vi "CheckDriveStatus.vi"(2 "Channel Properties":T1={"Channel Name"="", "Vel. Default"=5.0, "Acc. Default"=5.0, "Vel. Max"=5.0, "Vel. Min"=5.0, "Acc. Max"=5.0, "Acc. Min"=5.0, "Pulses/unit"=0.0, "Address"=0, "Pulse Offset"=0, "Pos Tolerance"=0.0, "Pulses/rev"=0.0, "Backlash/Eng units"=0.0, "Current Pos"=0.0, "Ch Status"=enum."Active", "Port Name"="", "Axis Transform mode"="", "Metadata Ch Name"="", "Type"=""} {"Current Pos" format="%.2f"; "Backlash/Eng units" format="%.2f"; "Pulses/rev" format="%.2f"; "Pos Tolerance" format="%.2f"; "Pulses/unit" format="%.2f"; "Acc. Min" format="%.2f"; "Acc. Max" format="%.2f"; "Vel. Min" format="%.2f"; "Vel. Max" format="%.2f"; "Acc. Default" format="%.2f"; "Vel. Default" format="%.2f"}, 3 "Axis info cluster":T2) -> (0 "Error string":string, 1 "Axis info cluster Out":T2)   [LabVIEW 2012]
uses:
  DriveStatus.ctl
  DriveProperties.ctl
  GenericDriveCommand.ctl
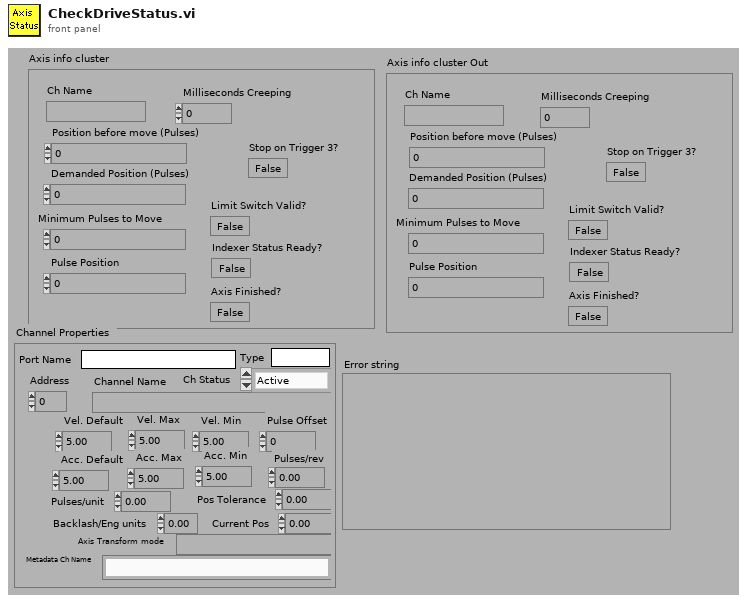
[diagram p1: front panel]
types:
  T1 = typedef "DriveProperties.ctl" = cluster{"Channel Name":string, "Vel. Default":dbl, "Acc. Default":dbl, "Vel. Max":dbl, "Vel. Min":dbl, "Acc. Max":dbl, "Acc. Min":dbl, "Pulses/unit":dbl, "Address":u8, "Pulse Offset":i32, "Pos Tolerance":dbl, "Pulses/rev":dbl, "Backlash/Eng units":dbl, "Current Pos":dbl, "Ch Status":enum16{"Active", "Offline", "Simulate"}, "Port Name":string, "Axis Transform mode":string, "Metadata Ch Name":string, "Type":string}
  T2 = typedef "DriveStatus.ctl" = cluster{"Ch Name":string, "Position before move (Pulses)":dbl, "Demanded Position (Pulses)":dbl, "Minimum Pulses to Move":dbl, "Pulse Position":dbl, "Indexer Status Ready?":bool, "Axis Finished?":bool, "Limit Switch Valid?":bool, "Milliseconds Creeping":u32, "Stop on Trigger 3?":bool}
  T3 = typedef "GenericDriveCommand.ctl" = string
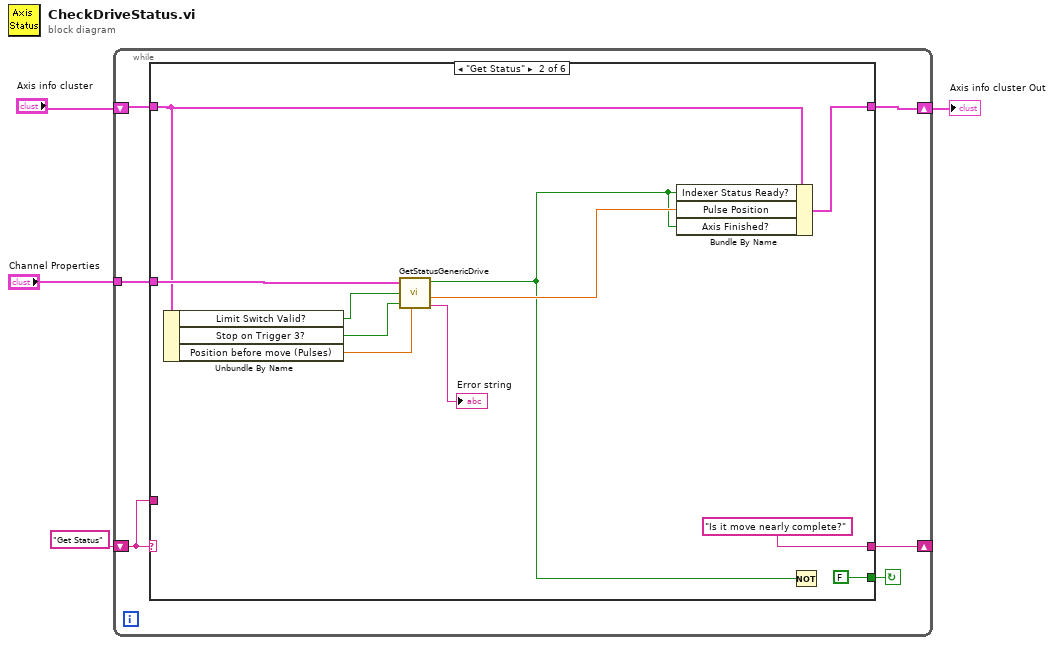
[diagram p0: block diagram]
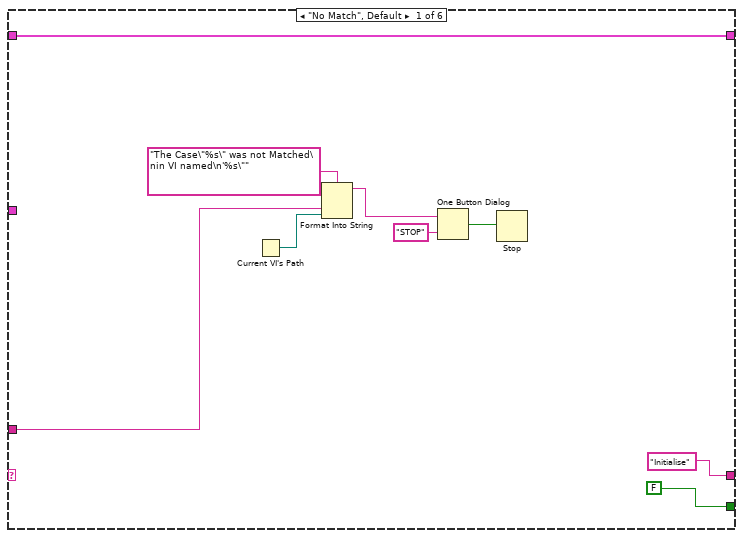
[diagram p2: hidden frame]
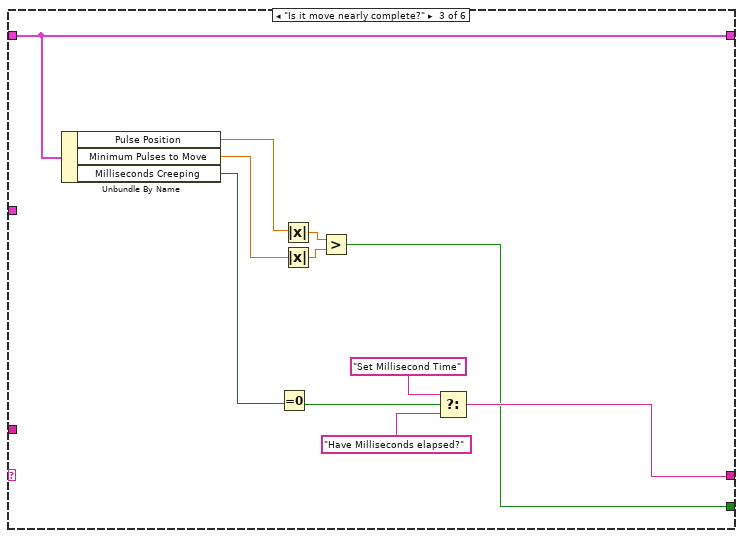
[diagram p3: hidden frame]
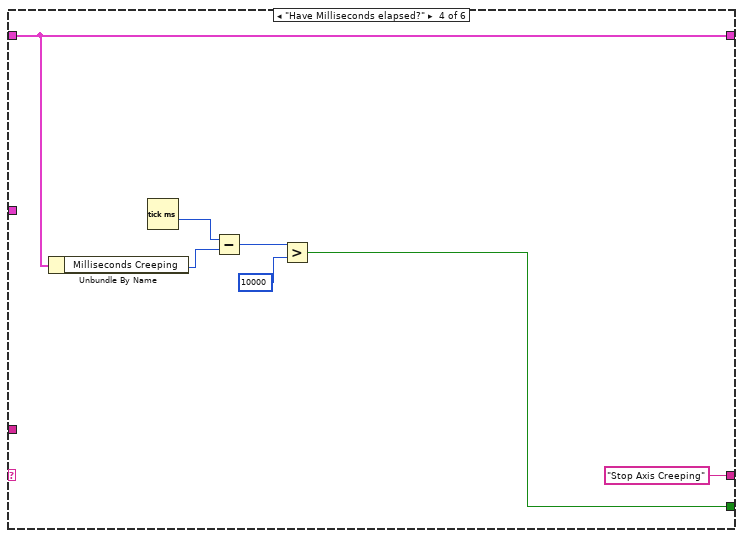
[diagram p4: hidden frame]
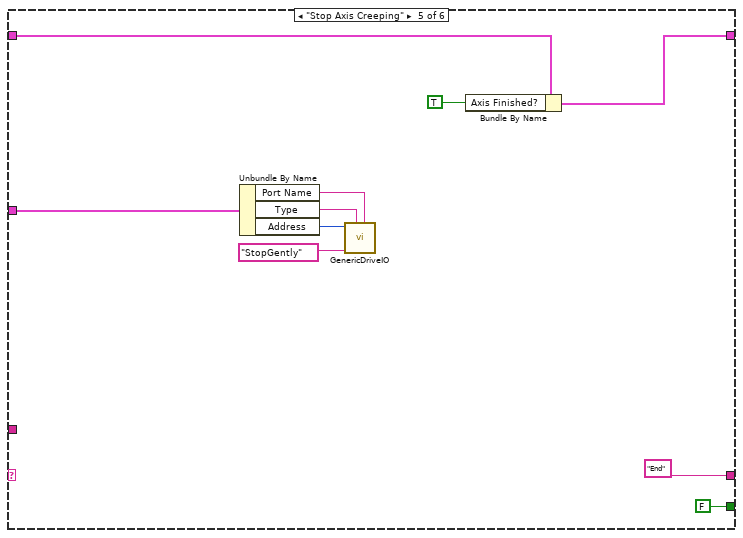
[diagram p5: hidden frame]
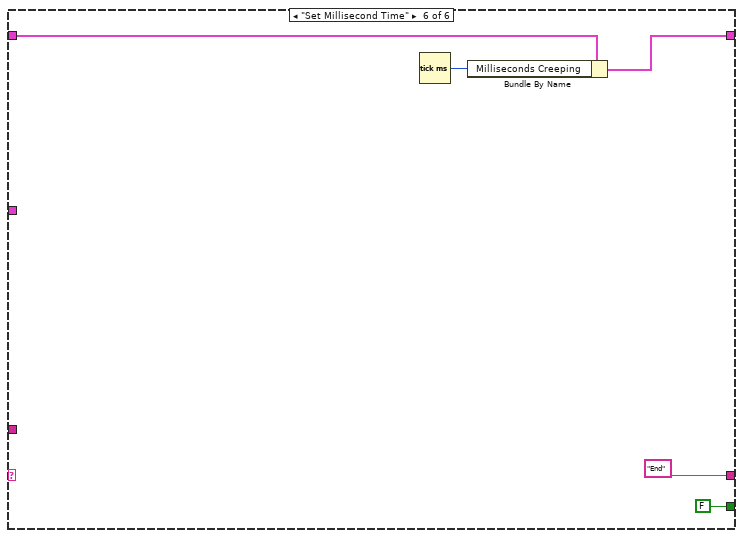
[diagram p6: hidden frame]
diagram:
  n1 = while {
    tunnel: "Channel Properties" -> [w6]
    shift-left: "Axis info cluster" -> [w7]
    shift-right: [w5] -> w2
    shift-left: "Get Status" -> [w8]
    shift-right: [w9] -> _
    stop <- w10 continue-if-true
    n2 = case shown="\"Get Status\"" w8 {
      tunnel: [FALSE FALSE w31 w42 FALSE FALSE] -> w10
      tunnel: ["Initialise" "Is it move nearly complete?" w32 "Stop Axis Creeping" "End" "End"] -> w9
      tunnel: w8 -> [w14 _ _ _ _ _]
      tunnel: w7 -> [w11 w27 w37 w47 w56 w62]
      tunnel: w6 -> [_ w29 _ _ w53 _]
      tunnel: [w11 w28 w37 w47 w55 w61] -> w5
      frame "No Match", Default {
        n3 = Current VI's Path() -> (path=w13:path)
        n4 = Format Into String(format string="The Case\"%s\" was not Matched\nin VI named\n'%s\"" ("Format String"), w14, w13) -> (resulting string=w17:string)  [unwired: 2 in, 1 out]
        n5 = One Button Dialog(message=w17, button name ("OK")="STOP") -> (true=w15:bool)
        n6 = Stop(stop? (T)=w15) -> ()
      }
      frame "Get Status" {
        n7 = Unbundle By Name(w27) -> ("Limit Switch Valid?"=w26:bool, "Stop on Trigger 3?"=w24:bool, "Position before move (Pulses)"=w20:dbl)
        n8 = call "GetStatusGenericDrive.vi"("Channel Properties"=w29, "Limit switch valid?"=w26, "Stop on Trigger 3?"=w24, "Position before move (Pulses)"=w20) -> ("Ready"=w22:bool, "Current Pulse Position"=w23:dbl, "Error string"=→"Error string":string)  [unwired: 2 out]
        n9 = Bundle By Name(cluster=w27, "Indexer Status Ready?"=w22, "Pulse Position"=w23, "Axis Finished?"=w22) -> (w28:T2)
        n10 = Not(x=w22) -> ()  [unwired: 1 out]
      }
      frame "Is it move nearly complete?" {
        n11 = Unbundle By Name(w37) -> ("Pulse Position"=w39:dbl, "Minimum Pulses to Move"=w38:dbl, "Milliseconds Creeping"=w36:u32)
        n12 = Equal To 0?(x=w36) -> (x = 0?=w35:bool)
        n13 = Absolute Value(x=w39) -> (abs(x)=w40:dbl)
        n14 = Absolute Value(x=w38) -> (abs(x)=w41:dbl)
        n15 = Greater?(x=w40, y=w41) -> (0:w31:bool)
        n16 = Select(t="Set Millisecond Time", s=w35, f="Have Milliseconds elapsed?") -> (s? t:f=w32:string)
      }
      frame "Have Milliseconds elapsed?" {
        n17 = Unbundle By Name(w47) -> ("Milliseconds Creeping"=w45:u32)
        n18 = Tick Count (ms)() -> (millisecond timer value=w46:u32)
        n19 = Subtract(x=w46, y=w45) -> (x-y=w44:u32)
        n20 = Greater?(x=w44, y=u32 10000) -> (0:w42:bool)
      }
      frame "Stop Axis Creeping" {
        n21 = Unbundle By Name(w53) -> ("Port Name"=w50:string, "Type"=w51:string, "Address"=w52:u8)
        n22 = call "GenericDriveIO.vi"("GenericDriveCommand"=T3 "StopGently", "Address"=w52, "Type"=w51, "Port Name"=w50) -> ()  [unwired: 2 in, 6 out]
        n23 = Bundle By Name(cluster=w56, "Axis Finished?"=TRUE) -> (w55:T2)
      }
      frame "Set Millisecond Time" {
        n24 = Tick Count (ms)() -> (millisecond timer value=w60:u32)
        n25 = Bundle By Name(cluster=w62, "Milliseconds Creeping"=w60) -> (w61:T2)
      }
    }
  }
  "Axis info cluster Out" <- w2
